vi "Parse Response (JSON).vi"(8 "error in":errorcluster, 10 "Response String In":string) -> (0 "error out":errorcluster, 1 "LabVIEW Error?":bool=TRUE, 2 "JSON out":refnum<class "JSON Null.lvclass">)   [LabVIEW 2015, in "JSONRPC Server.lvclass"]
uses:
  JSONRPC Server.lvclass
  <vilib>/National Instruments/JSON Support for LabVIEW/JSON Data Classes/JSON Datatype/JSON Null.lvclass
  <vilib>/National Instruments/JSON Support for LabVIEW/JSON Data Classes/JSON Helper/Parsing/Parse Value.vi
  <vilib>/National Instruments/JSON Support for LabVIEW/JSON Data Classes/JSON Helper/To More Specific Type (Object).vi
  <vilib>/National Instruments/JSON Support for LabVIEW/JSON Data Classes/JSON Object/Get Value (JSON).vi
  <vilib>/National Instruments/JSON Support for LabVIEW/JSON Data Classes/JSON Helper/To More Specific Type (Numeric).vi
  <vilib>/National Instruments/JSON Support for LabVIEW/JSON Data Classes/JSON Numeric/Read value (Numeric).vi
  <vilib>/National Instruments/JSON Support for LabVIEW/JSON Data Classes/JSON Helper/To More Specific Type (String).vi
  <vilib>/National Instruments/JSON Support for LabVIEW/JSON Data Classes/JSON String/Read value (String).vi
  <vilib>/National Instruments/JSON Support for LabVIEW/JSON Data Classes/JSON Helper/JSON Helper.lvclass
  <vilib>/National Instruments/JSON Support for LabVIEW/JSON Data Classes/JSON Basic Type/JSON Literal.lvclass
  <vilib>/National Instruments/JSON Support for LabVIEW/JSON Data Classes/JSON Numeric/JSON Numeric.lvclass
  <vilib>/National Instruments/JSON Support for LabVIEW/JSON Data Classes/JSON String/JSON String.lvclass
  <vilib>/National Instruments/JSON Support for LabVIEW/JSON Data Classes/JSON Object/JSON Object.lvclass
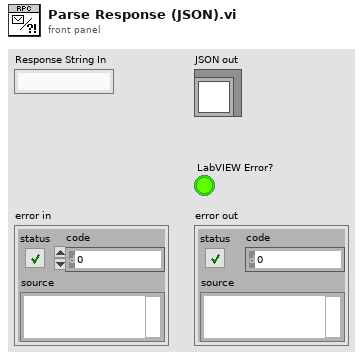
[diagram p1: front panel]
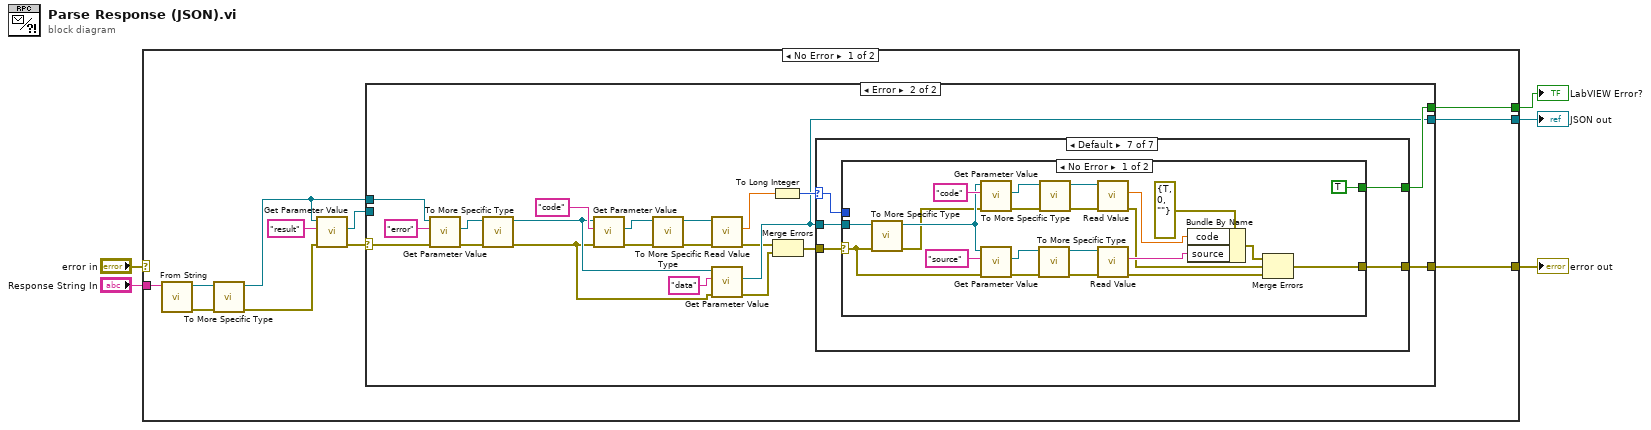
[diagram p0: block diagram]
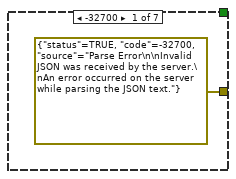
[diagram p3: hidden frame]
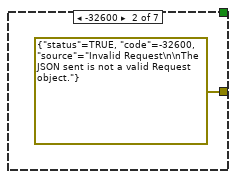
[diagram p4: hidden frame]
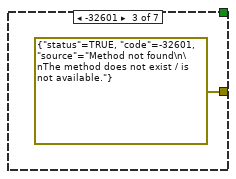
[diagram p5: hidden frame]
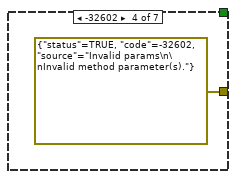
[diagram p6: hidden frame]
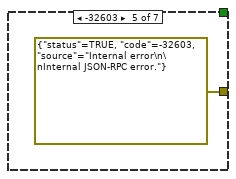
[diagram p7: hidden frame]
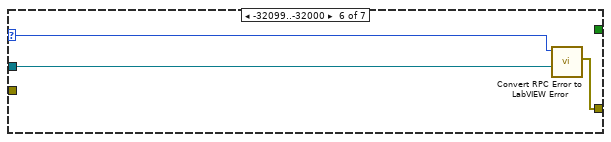
[diagram p8: hidden frame]
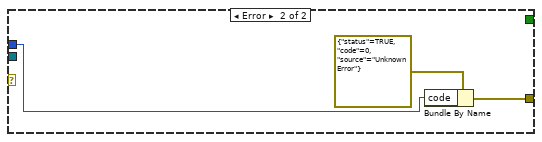
[diagram p9: hidden frame]
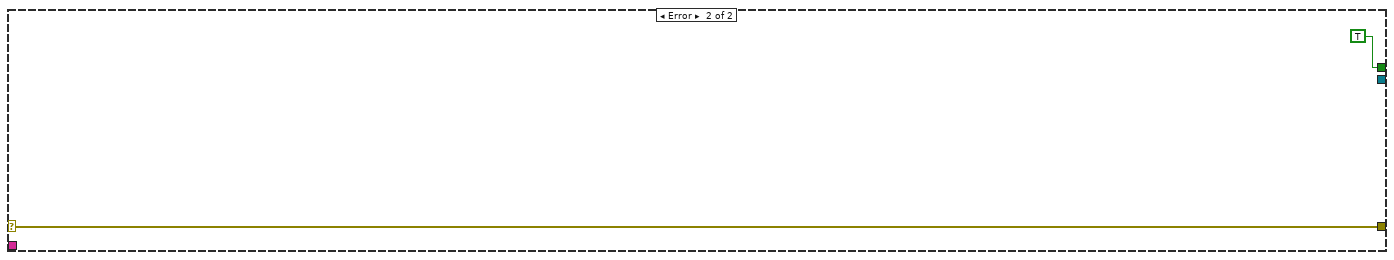
[diagram p10: hidden frame]
diagram:
  n1 = case shown="No Error" "error in" {
    selector: "error in" -> [_ w78]
    tunnel: "Response String In" -> [w13 _]
    tunnel: [w16 _] -> w1
    tunnel: [w15 w78] -> w3
    tunnel: [w14 TRUE] -> w2
    frame No Error {
      n2 = call <vilib>:"From String.vi"("JSON String"=w13) -> ("error out"=w12:errorcluster, "JSON out"=w11:refnum<class "JSON Null.lvclass">)  [unwired: 9 in]
      n3 = call-poly <vilib>:"To More Specific Type.vi"("error in (no error)"=w12, "JSON Datatype in"=w11) -> ("error out"=w9:errorcluster, "JSON Datatype out"=w8:refnum<class "JSON Object.lvclass">)  [unwired: 8 in]
      n4 = call-poly <vilib>:"Get Parameter Value.vi"("error in (no error)"=w9, "key"="result", "JSON Object in"=w8) -> ("error out"=w6:errorcluster, "value"=w7:refnum<class "JSON Null.lvclass">)  [unwired: 7 in]
      n5 = case shown="Error" w6 {
        selector: w6 -> [w17 w26]
        tunnel: [w18 w31] -> w16
        tunnel: [w17 w38] -> w15
        tunnel: [_ w37] -> w14
        tunnel: w8 -> [_ w36]
        tunnel: w7 -> [w18 _]
        frame No Error {
        }
        frame Error {
          n6 = call-poly <vilib>:"Get Parameter Value.vi"("error in (no error)"=w26, "key"="error", "JSON Object in"=w36) -> ("error out"=w25:errorcluster, "value"=w34:refnum<class "JSON Null.lvclass">)  [unwired: 7 in]
          n7 = call-poly <vilib>:"To More Specific Type.vi"("error in (no error)"=w25, "JSON Datatype in"=w34) -> ("error out"=w22:errorcluster, "JSON Datatype out"=w28:refnum<class "JSON Object.lvclass">)  [unwired: 8 in]
          n8 = call-poly <vilib>:"Get Parameter Value.vi"("error in (no error)"=w22, "key"="code", "JSON Object in"=w28) -> ("error out"=w24:errorcluster, "value"=w29:refnum<class "JSON Null.lvclass">)  [unwired: 7 in]
          n9 = call-poly <vilib>:"To More Specific Type.vi"("error in (no error)"=w24, "JSON Datatype in"=w29) -> ("error out"=w23:errorcluster, "JSON Numeric out"=w30:refnum<class "JSON Numeric.lvclass">)  [unwired: 8 in]
          n10 = call-poly <vilib>:"Read Value.vi"("error in (no error)"=w23, "JSON String in"=w30) -> ("error out"=w21:errorcluster, "value"=w27:dbl)  [unwired: 8 in]
          n11 = call-poly <vilib>:"Get Parameter Value.vi"("error in (no error)"=w22, "key"="data", "JSON Object in"=w28) -> ("error out"=w20:errorcluster, "value"=w31:refnum<class "JSON Null.lvclass">)  [unwired: 7 in]
          n12 = To Long Integer(number=w27) -> (32bit integer=w39:i32)
          n13 = Merge Errors(w21, w20) -> (w19:errorcluster)
          n14 = case shown="Default" w39 {
            selector: w39 -> [_ _ _ _ _ w47 w50]
            tunnel: [errorcluster {"status"=TRUE, "code"=-32700, "source"="Parse Error\n\nInvalid JSON was received by the server.\nAn error occurred on the server while parsing the JSON text."} ("error constant") errorcluster {"status"=TRUE, "code"=-32600, "source"="Invalid Request\n\nThe JSON sent is not a valid Request object."} ("error constant") errorcluster {"status"=TRUE, "code"=-32601, "source"="Method not found\n\nThe method does not exist / is not available."} ("error constant") errorcluster {"status"=TRUE, "code"=-32602, "source"="Invalid params\n\nInvalid method parameter(s)."} ("error constant") errorcluster {"status"=TRUE, "code"=-32603, "source"="Internal error\n\nInternal JSON-RPC error."} ("error constant") w45 w52] -> w38
            tunnel: w31 -> [_ _ _ _ _ w46 w51]
            tunnel: [_ _ _ _ _ _ w49] -> w37
            tunnel: w19 -> [_ _ _ _ _ _ w48]
            frame -32700 {
            }
            frame -32600 {
            }
            frame -32601 {
            }
            frame -32602 {
            }
            frame -32603 {
            }
            frame -32099..-32000 {
              n15 = call "Convert RPC Error to LabVIEW Error.vi"("JSON in"=w46, "RPC Error Code"=w47) -> ("error out"=w45:errorcluster)  [unwired: 9 in]
            }
            frame Default {
              n16 = case shown="No Error" w48 {
                selector: w48 -> [w57 _]
                tunnel: [w53 w75] -> w52
                tunnel: w51 -> [w72 _]
                tunnel: w50 -> [_ w76]
                tunnel: [TRUE _] -> w49
                frame No Error {
                  n17 = call-poly <vilib>:"To More Specific Type.vi"("error in (no error)"=w57, "JSON Datatype in"=w72) -> ("error out"=w62:errorcluster, "JSON Datatype out"=w65:refnum<class "JSON Object.lvclass">)  [unwired: 8 in]
                  n18 = call-poly <vilib>:"Get Parameter Value.vi"("error in (no error)"=w62, "key"="code", "JSON Object in"=w65) -> ("error out"=w61:errorcluster, "value"=w71:refnum<class "JSON Null.lvclass">)  [unwired: 7 in]
                  n19 = call-poly <vilib>:"Get Parameter Value.vi"("error in (no error)"=w57, "key"="source" ("Parameter Name"), "JSON Object in"=w65) -> ("error out"=w59:errorcluster, "value"=w66:refnum<class "JSON Null.lvclass">)  [unwired: 7 in]
                  n20 = call-poly <vilib>:"To More Specific Type.vi"("error in (no error)"=w59, "JSON Datatype in"=w66) -> ("error out"=w58:errorcluster, "JSON Datatype out"=w67:refnum<class "JSON String.lvclass">)  [unwired: 8 in]
                  n21 = call-poly <vilib>:"To More Specific Type.vi"("error in (no error)"=w61, "JSON Datatype in"=w71) -> ("error out"=w60:errorcluster, "JSON Numeric out"=w70:refnum<class "JSON Numeric.lvclass">)  [unwired: 8 in]
                  n22 = call-poly <vilib>:"Read Value.vi"("error in (no error)"=w60, "JSON String in"=w70) -> ("error out"=w56:errorcluster, "value"=w68:dbl)  [unwired: 8 in]
                  n23 = call-poly <vilib>:"Read Value.vi"("error in (no error)"=w58, "JSON String in"=w67) -> ("error out"=w55:errorcluster, "value"=w63:string)  [unwired: 8 in]
                  n24 = Bundle By Name(cluster=errorcluster {"status"=TRUE, "code"=0, "source"=""} ("error constant"), "code"=w68, "source"=w63) -> (w54:errorcluster)
                  n25 = Merge Errors(w54, w56, w55) -> (w53:errorcluster)
                }
                frame Error {
                  n26 = Bundle By Name(cluster=errorcluster {"status"=TRUE, "code"=0, "source"="Unknown Error"} ("error constant"), "code"=w76) -> (w75:errorcluster)
                }
              }
            }
          }
        }
      }
    }
    frame Error {
    }
  }
  "error out" <- w3
  "JSON out" <- w1
  "LabVIEW Error?" <- w2
